vi "关键参数交互.vi"(9 "量程下拉列表":refnum<vi>, 10 "测量模式下拉列表":refnum<vi>, 11 "测量参数":refnum<vi>) -> ()   [LabVIEW 2016, in "斯坦道总磷.lvlib"]
panel:
  out "x != y?":T1
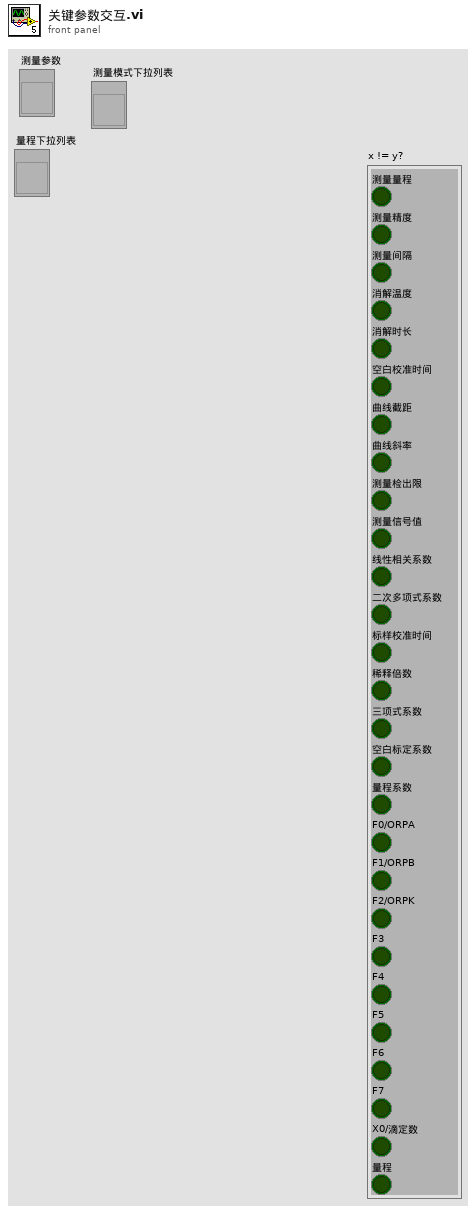
[diagram p1: front panel]
types:
  T1 = cluster{"测量量程":bool, "测量精度":bool, "测量间隔":bool, "消解温度":bool, "消解时长":bool, "空白校准时间":bool, "曲线截距":bool, "曲线斜率":bool, "测量检出限":bool, "测量信号值":bool, "线性相关系数":bool, "二次多项式系数":bool, "标样校准时间":bool, "稀释倍数":bool, "三项式系数":bool, "空白标定系数":bool, "量程系数":bool, "F0/ORPA":bool, "F1/ORPB":bool, "F2/ORPK":bool, "F3":bool, "F4":bool, "F5":bool, "F6":bool, "F7":bool, "X0/滴定数":bool, "量程":bool}
  T2 = cluster{"chose":string, "公式":cluster{"X^2":dbl, "X":dbl, "b":dbl}}
  T3 = cluster{"测量量程":dbl, "测量精度":dbl, "测量间隔":dbl, "消解温度":dbl, "消解时长":dbl, "空白校准时间":timestamp, "曲线截距":dbl, "曲线斜率":dbl, "测量检出限":dbl, "测量信号值":dbl, "线性相关系数":dbl, "二次多项式系数":dbl, "标样校准时间":timestamp, "稀释倍数":dbl, "三项式系数":dbl, "空白标定系数":dbl, "量程系数":dbl, "F0/ORPA":dbl, "F1/ORPB":dbl, "F2/ORPK":dbl, "F3":dbl, "F4":dbl, "F5":dbl, "F6":dbl, "F7":dbl, "X0/滴定数":dbl, "量程":dbl}
  T4 = cluster{"时间标识":timestamp, "设备":string, "日志信息":string, "流程参数":string}
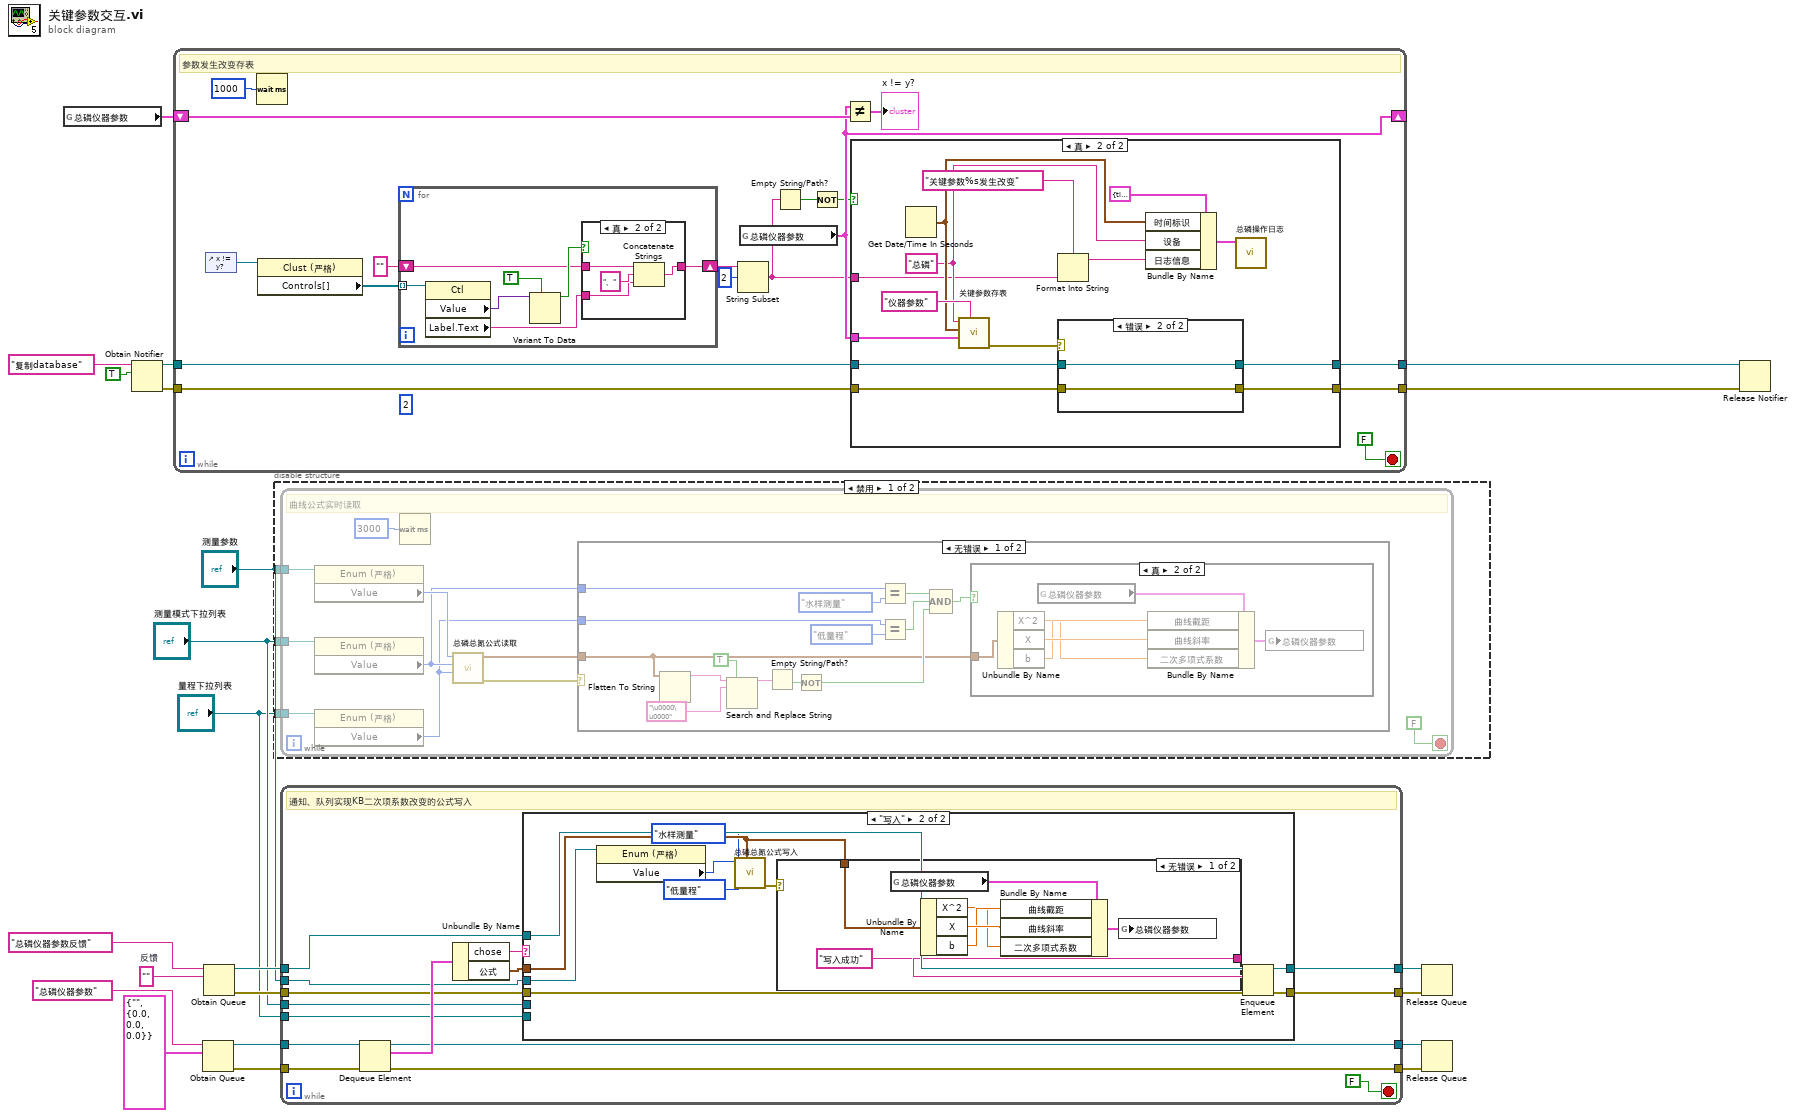
[diagram p0: block diagram]
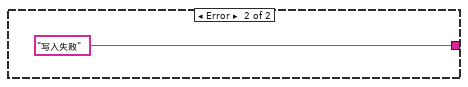
[diagram p6: hidden frame]
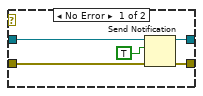
[diagram p9: hidden frame]
diagram:
  w13 = ""  # 反馈
  n1 = global read "总磷断电保存全局变量.vi" "总磷仪器参数"() -> (w22:T3)
  n2 = Obtain Notifier(name (unnamed)="复制database" ("名称（未命名）"), notification data type=TRUE) -> (notifier out=w7:refnum<notifier>, error out=w6:errorcluster)  [unwired: 2 in, 1 out]
  n3 = while {
    shift-right: [w34] -> _
    shift-left: w22 -> [w37]
    tunnel: w7 -> [w33]
    tunnel: w6 -> [w32]
    tunnel: [w31] -> w5
    tunnel: [w30] -> w4
    stop <- FALSE stop-if-true
    (unwired) 2 ("偏移量(0)")
    # "参数发生改变存表"
    n4 = control-ref of="x != y?"() -> (w35:refnum<vi>)
    n5 = Wait (ms)(milliseconds to wait=u32 1000 ("等待时间（毫秒）")) -> ()  [unwired: 1 out]
    n6 = property class="Clust (严格)"(reference=w35) -> ("Controls[]"=w26:refnum<vi>[])  [unwired: 1 in, 2 out]
    n7 = for {
      tunnel: w26 -> [w46] mode=indexing
      shift-right: [w40] -> w28
      shift-left: "" -> [w42]
      n8 = property class="Ctl"(reference=w46) -> ("Value"=w44:variant, "Label.Text"=w41:string)  [unwired: 1 in, 2 out]
      n9 = Variant To Data(type=TRUE, Variant=w44) -> (data=w43:bool)  [unwired: 1 in, 1 out]
      n10 = case shown="真" w43 {
        tunnel: w42 -> [w47 w51]
        tunnel: w41 -> [_ w48]
        tunnel: [w47 w50] -> w40
        frame False {
        }
        frame True {
          n11 = Concatenate Strings(w51, "、", w48) -> (w50:string)
        }
      }
    }
    n12 = String Subset(string=w28, offset (0)=2 ("偏移量(0)")) -> (substring=w24:string)  [unwired: 1 in]
    n13 = global read "总磷断电保存全局变量.vi" "总磷仪器参数"() -> (w34:T3)
    n14 = Empty String/Path?(string/path=w24) -> (empty?=w29:bool)
    n15 = Not(x=w29) -> (.not. x?=w25:bool)
    n16 = Not Equal?(x=w34, y=w37) -> (x != y?=→"x != y?":T1)
    n17 = case shown="真" w25 {
      tunnel: w34 -> [_ w66]
      tunnel: w24 -> [_ w60]
      tunnel: w33 -> [w52 w58]
      tunnel: w32 -> [w53 w57]
      tunnel: [w52 w56] -> w31
      tunnel: [w53 w55] -> w30
      frame False {
      }
      frame True {
        w62 = "总磷" ("仪器名称")
        n18 = Get Date/Time In Seconds() -> (seconds since 1Jan1904=w63:timestamp)
        n19 = call "关键参数存表.vi"("table"="仪器参数", "仪器参数"=w66, "datatime"=w63, "仪器名称"=w62) -> ("error out"=w54:errorcluster)  [unwired: 7 in]
        n20 = Format Into String(format string="关键参数%s发生改变" ("格式字符串"), w60) -> (resulting string=w59:string)  [unwired: 2 in, 1 out]
        n21 = case shown="错误" w54 {
          tunnel: w58 -> [w72 w74]
          tunnel: w57 -> [w71 w73]
          tunnel: [w69 w74] -> w56
          tunnel: [w68 w73] -> w55
          frame No Error {
            n22 = Send Notification(notification=TRUE ("通知"), notifier=w72, error in (no error)=w71) -> (notifier out=w69:refnum<notifier>, error out=w68:errorcluster)
          }
          frame Error {
          }
        }
        n23 = Bundle By Name(cluster=T4 {"时间标识"=timestamp(0 s since 1904-01-01), "设备"="", "日志信息"="", "流程参数"=""} ("data in"), "时间标识"=w63, "设备"=w62, "日志信息"=w59) -> (w64:T4)
        n24 = call "总磷操作日志.vi"("data in"=w64) -> ()  [unwired: 11 in]
      }
    }
  }
  n25 = Obtain Queue(name (unnamed)="总磷仪器参数" ("名称（未命名）"), element data type=T2 {"chose"="", "公式"={"X^2"=0.0, "X"=0.0, "b"=0.0}}) -> (queue out=w21:refnum<queue>, error out=w20:errorcluster)  [unwired: 3 in, 1 out]
  n26 = Obtain Queue(name (unnamed)="总磷仪器参数反馈" ("名称（未命名）"), element data type=w13) -> (queue out=w14:refnum<queue>, error out=w12:errorcluster)  [unwired: 3 in, 1 out]
  n27 = disable-structure shown="禁用" {
    disable-tunnel: "测量参数" -> [w77 _]
    disable-tunnel: "测量模式下拉列表" -> [w76 _]
    disable-tunnel: "量程下拉列表" -> [w75 _]
    frame Disabled {
      n28 = while {
        tunnel: w77 -> [w85]
        tunnel: w76 -> [w84]
        tunnel: w75 -> [w83]
        stop <- FALSE stop-if-true
        # "曲线公式实时读取"
        n29 = property class="Enum (严格)"(reference=w85) -> ("Value"=w82:enum16{"总磷", "总氮"})  [unwired: 1 in, 2 out]
        n30 = property class="Enum (严格)"(reference=w84) -> ("Value"=w81:enum16{"水样测量", "零点核查", "跨度核查", "标样核查", "加标回收"})  [unwired: 1 in, 2 out]
        n31 = property class="Enum (严格)"(reference=w83) -> ("Value"=w80:enum16{"低量程", "高量程"})  [unwired: 1 in, 2 out]
        n32 = Wait (ms)(milliseconds to wait=u32 3000 ("等待时间（毫秒）")) -> ()  [unwired: 1 out]
        n33 = call "总磷总氮公式读取.vi"("量程"=w80, "测量模式"=w81, "测量参数"=w82) -> ("error out"=w78:errorcluster, "公式"=w79:cluster{"X^2":dbl, "X":dbl, "b":dbl})  [unwired: 7 in]
        n34 = case shown="无错误" w78 {
          tunnel: w81 -> [w101 _]
          tunnel: w79 -> [w88 _]
          tunnel: w80 -> [w95 _]
          frame No Error {
            n35 = Flatten To String(anything=w88) -> (data string=w94:string)  [unwired: 3 in, 2 out]
            n36 = Search and Replace String(replace all?=TRUE ("替换全部？(F)"), input string=w94, search string="\u0000\u0000" ("数据字符串")) -> (result string=w92:string)  [unwired: 5 in, 3 out]
            n37 = Empty String/Path?(string/path=w92) -> (empty?=w91:bool)
            n38 = Not(x=w91) -> (.not. x?=w89:bool)
            n39 = Equal?(x=w101, y=enum16{"水样测量", "零点核查", "跨度核查", "标样核查", "加标回收"}."水样测量") -> (x = y?=w98:bool)
            n40 = Equal?(x=w95, y=enum16{"低量程", "高量程"}."低量程") -> (x = y?=w97:bool)
            n41 = Compound Arithmetic op=AND ("复合运算")(w98, w97, w89) -> (w96:bool)
            n42 = case shown="真" w96 {
              tunnel: w88 -> [_ w107]
              frame False {
              }
              frame True {
                n43 = Unbundle By Name(w107) -> ("X^2"=w104:dbl, "X"=w106:dbl, "b"=w105:dbl)
                n44 = global read "总磷断电保存全局变量.vi" "总磷仪器参数"() -> (w103:T3)
                n45 = Bundle By Name(cluster=w103, "曲线截距"=w105, "曲线斜率"=w106, "二次多项式系数"=w104) -> (w102:T3)
                n46 = global write "总磷断电保存全局变量.vi" "总磷仪器参数"(w102) -> ()
              }
            }
          }
          frame Error {
          }
        }
      }
    }
    frame Enabled {
    }
  }
  n47 = while {
    tunnel: w21 -> [w121]
    tunnel: w20 -> [w120]
    tunnel: [w116] -> w17
    tunnel: [w115] -> w16
    tunnel: w14 -> [w114]
    tunnel: w12 -> [w113]
    tunnel: [w112] -> w11
    tunnel: [w111] -> w10
    tunnel: "测量参数" -> [w110]
    tunnel: "测量模式下拉列表" -> [w109]
    tunnel: "量程下拉列表" -> [w108]
    stop <- FALSE stop-if-true
    # "通知、队列实现KB二次项系数改变的公式写入"
    n48 = Dequeue Element(queue=w121, error in (no error)=w120) -> (queue out=w116:refnum<queue>, element=w119:T2, error out=w115:errorcluster)  [unwired: 1 in, 1 out]
    n49 = Unbundle By Name(w119) -> ("chose"=w118:string, "公式"=w117:cluster{"X^2":dbl, "X":dbl, "b":dbl})
    n50 = case shown="\"写入\"" w118 {
      tunnel: w117 -> [_ w127]
      tunnel: w114 -> [w124 w134]
      tunnel: w113 -> [w123 w132]
      tunnel: [w124 w131] -> w112
      tunnel: [w123 w130] -> w111
      tunnel: w110 -> [_ w128]
      tunnel: w109 -> [_ _]
      tunnel: w108 -> [_ _]
      frame "假", Default {
      }
      frame "写入" {
        n51 = property class="Enum (严格)"(reference=w128) -> ("Value"=w129:enum16{"总磷", "总氮"})  [unwired: 1 in, 2 out]
        n52 = call "总磷总氮公式写入.vi"("公式"=w127, "量程"=enum16{"低量程", "高量程"}."低量程", "测量模式"=enum16{"水样测量", "零点核查", "跨度核查", "标样核查", "加标回收"}."水样测量", "测量参数"=w129) -> ("error out"=w135:errorcluster)  [unwired: 7 in]
        n53 = case shown="无错误" w135 {
          tunnel: ["写入成功" ("消息") "写入失败" ("消息")] -> w133
          tunnel: w127 -> [w136 _]
          frame No Error {
            n54 = global read "总磷断电保存全局变量.vi" "总磷仪器参数"() -> (w138:T3)
            n55 = Unbundle By Name(w136) -> ("X^2"=w139:dbl, "X"=w141:dbl, "b"=w140:dbl)
            n56 = Bundle By Name(cluster=w138, "曲线截距"=w140, "曲线斜率"=w141, "二次多项式系数"=w139) -> (w137:T3)
            n57 = global write "总磷断电保存全局变量.vi" "总磷仪器参数"(w137) -> ()
          }
          frame Error {
          }
        }
        n58 = Enqueue Element(queue=w134, element=w133, error in (no error)=w132) -> (queue out=w131:refnum<queue>, error out=w130:errorcluster)  [unwired: 1 in, 1 out]
      }
    }
  }
  n59 = Release Queue(queue=w11, error in (no error)=w10) -> ()  [unwired: 1 in, 3 out]
  n60 = Release Queue(queue=w17, error in (no error)=w16) -> ()  [unwired: 1 in, 3 out]
  n61 = Release Notifier(notifier=w5, error in (no error)=w4) -> ()  [unwired: 1 in, 3 out]
